vi "Record Assert Error.vi"   [LabVIEW 2023]
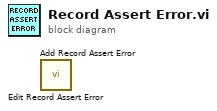
[diagram p0: block diagram]
diagram:
  n1 = call "Edit Record Assert Error.vi"() -> ()  [unwired: 10 in, 2 out]
  n2 = call "Add Record Assert Error.vi"() -> ()  [unwired: 10 in, 2 out]
